vi "Store The Settings.vi"(8 "Error In":errorcluster, 11 "Settings":refnum<class "Settings.lvclass">) -> (0 "Error Out":errorcluster)   [LabVIEW 2016, in "Error Manager.lvlib" / "Settings.lvclass"]
doc: "This VI stores the Settings object in a class variable."
uses:
  Settings.lvclass
  Settings (class variable).vi
panel:
  # "Development\nControls or indicators that are useful for development or testing, but which are not outputs of the VI."
  # "Input\nInputs to the VI"
  # "Output\nOutputs of the VI"
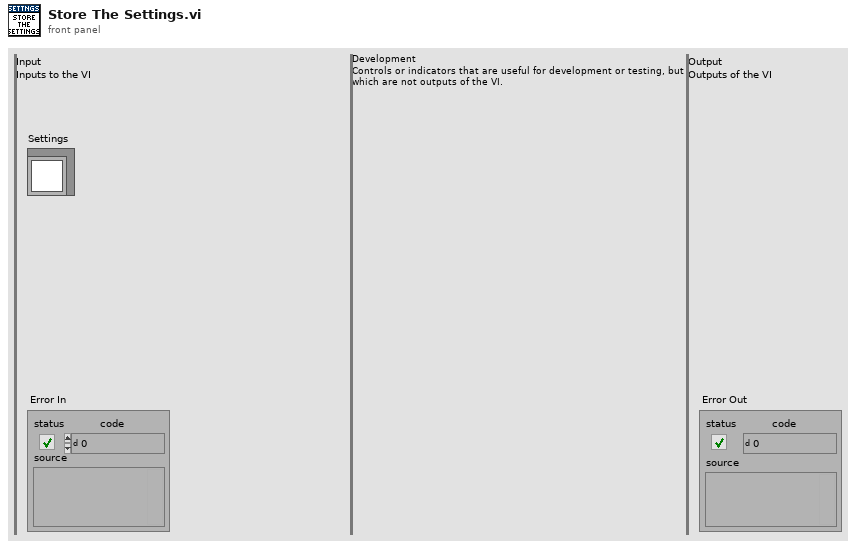
[diagram p1: front panel]
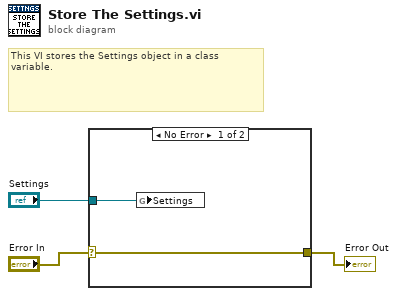
[diagram p0: block diagram]
diagram:
  # "This VI stores the Settings object in a class variable."
  n1 = case shown="No Error" "Error In" {
    selector: "Error In" -> [w5 w6]
    tunnel: [w5 w6] -> w2
    tunnel: "Settings" -> [w4 _]
    frame No Error {
      n2 = global write "Settings (class variable).vi" "Settings"(w4) -> ()
    }
    frame Error {
    }
  }
  "Error Out" <- w2
